vi "EPA Polynom Ordnung je Komponente für Protokoll.vi"(5 "Aktion":T3, 7 "error in (no error)":errorcluster caption="Fehler (Eingang, kein Fehler)", 9 "Index in":T1, 10 "EPA Optionsfeld":T2=enum."Rohwert") -> (0 "error out":errorcluster caption="Fehler (Ausgang)", 1 "EPA Optionsfelder out":T2[][](array[typedef]), 2 "Index out":T1, 3 "EPA Optionsfeld out":T2)   [LabVIEW 2020, in "Linearisierung v2.lvlib" / "Protokoll.lvlib"]
uses:
  Protokoll.lvlib
  EPA Optionsfeld.ctl
  Linearisierung v2.lvlib
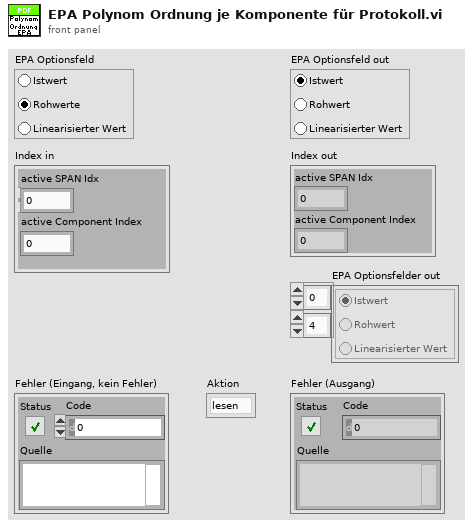
[diagram p1: front panel]
types:
  T1 = cluster{"active SPAN Idx":i32, "active Component Index":i32}
  T2 = typedef "Linearisierung v2.lvlib/EPA Optionsfeld.ctl" = enum32{"Istwert", "Rohwert", "Linearisierter Wert"}
  T3 = typedef "Linearisierung v2.lvlib/Protokoll.lvlib/Aktion EPA Polynom Ordnung je Komponente für Protokoll.ctl" = enum16{"lesen", "schreiben", "init", "init initial"}
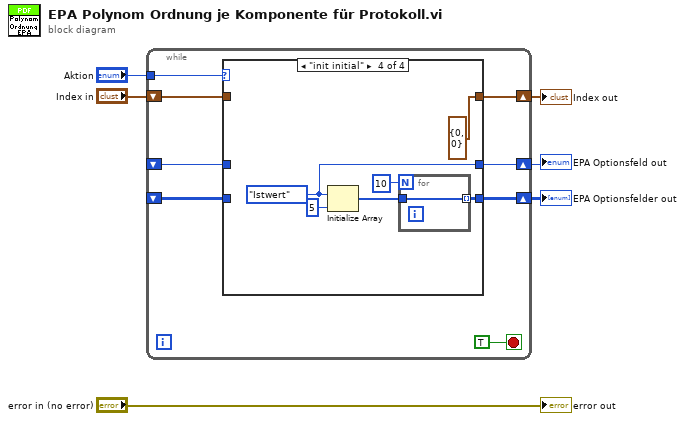
[diagram p0: block diagram]
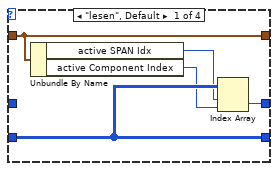
[diagram p2: hidden frame]
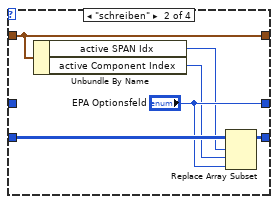
[diagram p3: hidden frame]
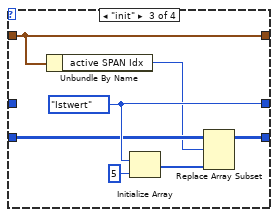
[diagram p4: hidden frame]
diagram:
  n1 = while {
    tunnel: "Aktion" -> [w13]
    shift-right: [w12] -> w5
    shift-left: "Index in" -> [w11]
    shift-right: [w10] -> w3
    shift-left: _ -> [w9]
    shift-right: [w8] -> w2
    shift-left: _ -> [w7]
    stop <- TRUE stop-if-true
    n2 = case shown="\"init initial\"" w13 {
      tunnel: [w17 w22 w30 T1 {"active SPAN Idx"=0, "active Component Index"=0} ("Index in")] -> w12
      tunnel: w11 -> [w17 w22 w30 _]
      tunnel: [w19 "EPA Optionsfeld" w31 w37] -> w10
      tunnel: w9 -> [_ _ _ _]
      tunnel: [w18 w24 w29 w33] -> w8
      tunnel: w7 -> [w18 w25 w28 _]
      frame "lesen", Default {
        n3 = Unbundle By Name(w17) -> ("active SPAN Idx"=w16:i32, "active Component Index"=w15:i32)
        n4 = Index Array(array=w18, index (row)=w16, index (col)=w15) -> (element=w19:T2)
      }
      frame "schreiben" {
        n5 = Unbundle By Name(w22) -> ("active SPAN Idx"=w21:i32, "active Component Index"=w20:i32)
        n6 = Replace Array Subset(array=w25, new element="EPA Optionsfeld", index (row)=w21, index (col)=w20) -> (w24:T2[][])
      }
      frame "init" {
        w31 = EPA_Optionsfeld."Istwert" ("EPA Optionsfeld")
        n7 = Unbundle By Name(w30) -> ("active SPAN Idx"=w27:i32)
        n8 = Initialize Array(w31, 5 ("Dimensionsgröße")) -> (w26:T2[])
        n9 = Replace Array Subset(array=w28, new element=w26, index (row)=w27) -> (w29:T2[][])  [unwired: 1 in]
      }
      frame "init initial" {
        w37 = EPA_Optionsfeld."Istwert" ("EPA Optionsfeld")
        n10 = Initialize Array(w37, 5 ("Dimensionsgröße")) -> (w34:T2[])
        n11 = for {
          N: 10 -> [_]
          tunnel: w34 -> [w39]
          tunnel: [w39] -> w33 mode=indexing
        }
      }
    }
  }
  "EPA Optionsfeld out" <- w3
  "EPA Optionsfelder out" <- w2
  "Index out" <- w5
  "error out" <- "error in (no error)"
